vi "Curtin1_Bands.vi"(5 "File Names":string[](array[string]), 9 "Bands":u16, 10 "Excel?":bool, 11 "Magnitude":cluster{dbl, "df":dbl, dbl[]}[](array[cluster])) -> (0 "Raw Data":T1, 3 "Filter":T2(array[cluster]))   [LabVIEW 2022 SP3]
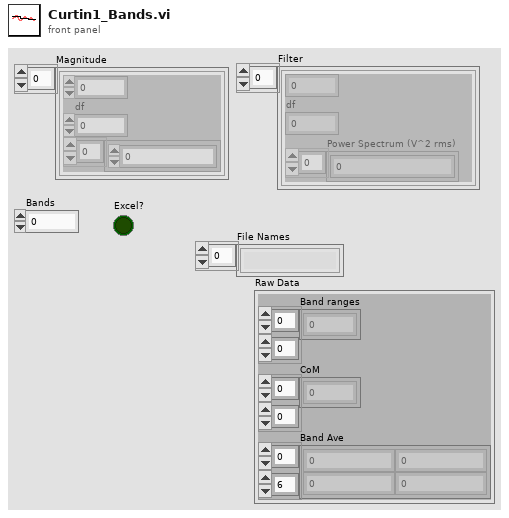
[diagram p1: front panel]
types:
  T1 = cluster{"Band ranges":dbl[][], "CoM":dbl[][], "Band Ave":dbl[][]}
  T2 = cluster{dbl, "df":dbl, "Power Spectrum (V^2 rms)":dbl[]}[]
  T3 = cluster{"Name":string, "Color":u32, "Style":u8, "Point Style":u8, "Name Visible":bool, "Allow Drag":bool, "Cursor Mode":u32, "Plot":i32, "Index":i32, "Position":cluster{"X":dbl, "Y":dbl}, "X Scale":u32, "Y Scale":u32, "Watch Plots":i32[], "Watch All Plots":bool, "Plot Area":i32, "Label Offset":cluster{"X":dbl, "Y":dbl}}[]
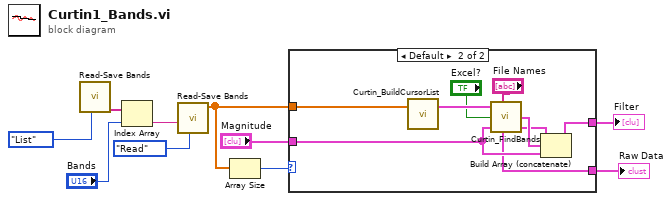
[diagram p0: block diagram]
diagram:
  n1 = call "Read-Save Bands.vi"("Task"=enum16{"Save", "Read", "List"}."List") -> ("file names"=w2:string[])  [unwired: 7 in, 3 out]
  n2 = Index Array(array=w2, index="Bands") -> (element=w1:string)
  n3 = call "Read-Save Bands.vi"("Task"=enum16{"Save", "Read", "List"}."Read", "Name"=w1) -> ("Frequencies"=w5:dbl[])  [unwired: 6 in, 3 out]
  n4 = Array Size(array=w5) -> (size(s)=w6:i32)
  n5 = case shown="Default" w6 {
    tunnel: w5 -> [_ w13]
    tunnel: "Magnitude" -> [w11 w14]
    tunnel: [w11 w19] -> w8
    tunnel: [_ w12] -> w3
    frame 0 {
    }
    frame Default {
      n6 = call "Curtin_BuildCursorList.vi"("Fctr"=w13) -> ("Cursor List"=w20:T3)  [unwired: 1 in, 1 out]
      n7 = call "Curtin_FindBands.vi"("CrsrList"=w20, "Labels"="File Names", "Excel?"="Excel?", "Magnitude"=w14) -> ("Raw Data"=w12:T1, "Filter"=w18:T2, "Centroids"=w17:T2)  [unwired: 1 out]
      n8 = Build Array (concatenate)(w17, w18, w14) -> (w19:T2)
    }
  }
  "Filter" <- w8
  "Raw Data" <- w3
